vi "List_Inst_Positions.vi"(1 "Position":T1(array[cluster]) {"Z" format="%.1f"; "Y" format="%.1f"; "X" format="%.1f"}) -> (0 "Position Info":string[][](array[string]))   [LabVIEW 2010]
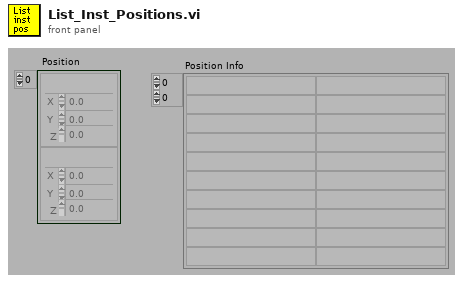
[diagram p1: front panel]
types:
  T1 = cluster{"Name":string, "X":dbl, "Y":dbl, "Z":dbl}[]
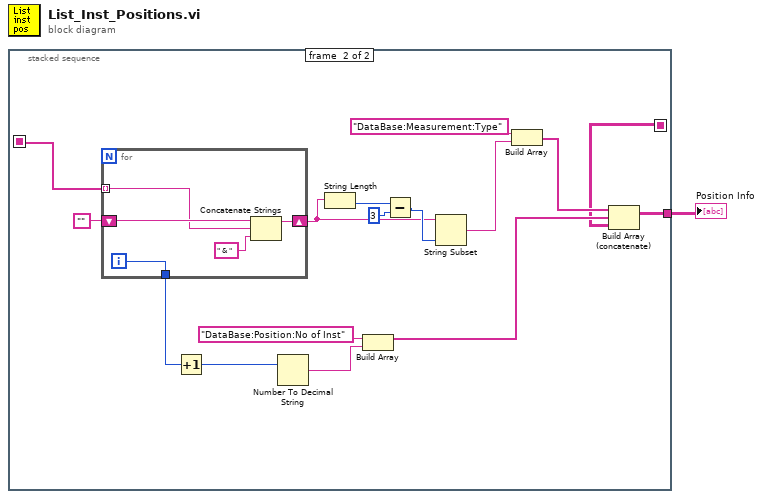
[diagram p0: block diagram]
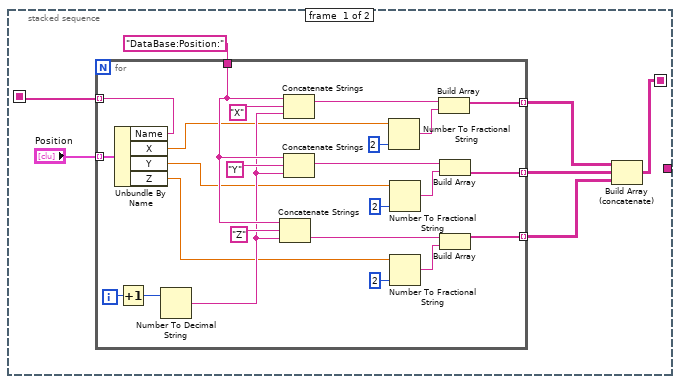
[diagram p2: hidden frame]
diagram:
  n1 = stacked-sequence {
    seq-local: [w4 _] -> [_ w34]
    seq-local: [w2 _] -> [_ w44]
    tunnel: [_ w33] -> w1
    frame #0 {
      n2 = for {
        tunnel: "Position" -> [w32] mode=indexing
        tunnel: "DataBase:Position:" -> [w29]
        tunnel: [w13] -> w7 mode=indexing
        tunnel: [w12] -> w6 mode=indexing
        tunnel: [w11] -> w5 mode=indexing
        tunnel: [w9] -> w2 mode=indexing
        i -> [w30]
        n3 = Unbundle By Name(w32) -> ("Name"=w9:string, "X"=w22:dbl, "Y"=w16:dbl, "Z"=w15:dbl)
        n4 = Increment(x=w30) -> (x+1=w10:i32)
        n5 = Number To Decimal String(number=w10) -> (decimal integer string=w26:string)  [unwired: 1 out]
        n6 = Concatenate Strings(w29, "Z", w26) -> (w14:string)
        n7 = Concatenate Strings(w29, "X", w26) -> (w25:string)
        n8 = Concatenate Strings(w29, "Y", w26) -> (w17:string)
        n9 = Number To Fractional String(number=w22, precision (6)=i16 2) -> (F-format string=w23:string)  [unwired: 2 out]
        n10 = Number To Fractional String(number=w16, precision (6)=i16 2) -> (F-format string=w21:string)  [unwired: 2 out]
        n11 = Number To Fractional String(number=w15, precision (6)=i16 2) -> (F-format string=w18:string)  [unwired: 2 out]
        n12 = Build Array(w25, w23) -> (w12:string[])
        n13 = Build Array(w17, w21) -> (w13:string[])
        n14 = Build Array(w14, w18) -> (w11:string[])
      }
      n15 = Build Array (concatenate)(w6, w7, w5) -> (w4:string[][])
    }
    frame #1 {
      n16 = for {
        shift-right: [w52] -> w40
        shift-left: "" -> [w53]
        tunnel: w44 -> [w51] mode=indexing
        tunnel: [w49] -> w38
        i -> [w49]
        n17 = Concatenate Strings(w53, w51, " & ") -> (w52:string)
      }
      n18 = Increment(x=w38) -> (x+1=w37:i32)
      n19 = Number To Decimal String(number=w37) -> (decimal integer string=w47:string)  [unwired: 1 out]
      n20 = String Length(string=w40) -> (length=w43:i32)
      n21 = Build Array("DataBase:Position:No of Inst", w47) -> (w35:string[])
      n22 = Subtract(x=w43, y=3) -> (x-y=w41:i32)
      n23 = String Subset(string=w40, length (rest)=w41) -> (substring=w39:string)  [unwired: 1 out]
      n24 = Build Array("DataBase:Measurement:Type", w39) -> (w36:string[])
      n25 = Build Array (concatenate)(w36, w35, w34) -> (w33:string[][])
    }
  }
  "Position Info" <- w1
